vi "Get Autonomous Data.vi"(11 "Autonomous Selectin":string="Robot Right Switch Left") -> (3 "Autonomous Data Selected":T1(array[cluster]))   [LabVIEW 2017]
uses:
  Framework/Robot Global Data.vi
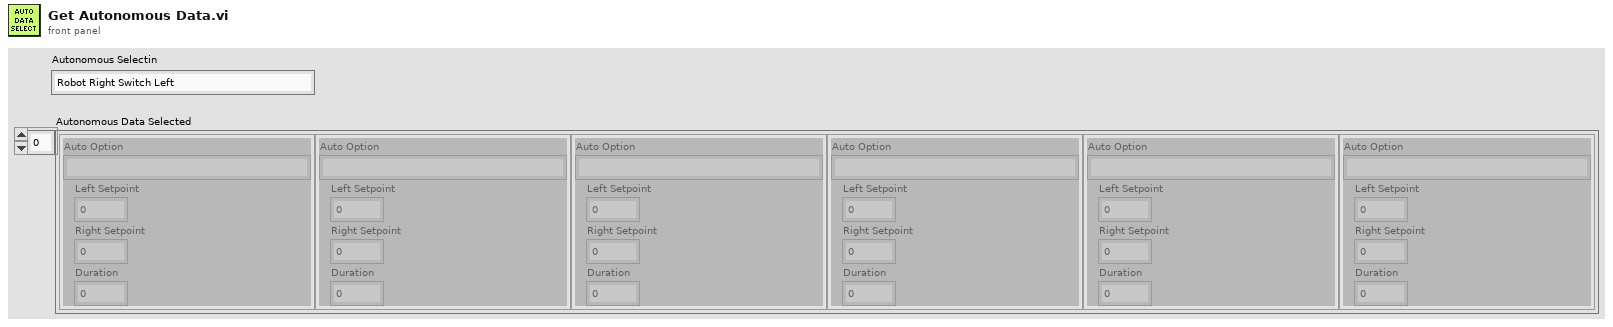
[diagram p1: front panel]
types:
  T1 = cluster{"Auto Option":string, "Left Setpoint":dbl, "Right Setpoint":dbl, "Duration":dbl}[]
  T2 = cluster{"Auto Option":string, "Left Setpoint":dbl, "Right Setpoint":dbl, "Duration":dbl}[][]
  T3 = cluster{"Auto Option":string, "Left Setpoint":dbl, "Right Setpoint":dbl, "Duration":dbl}
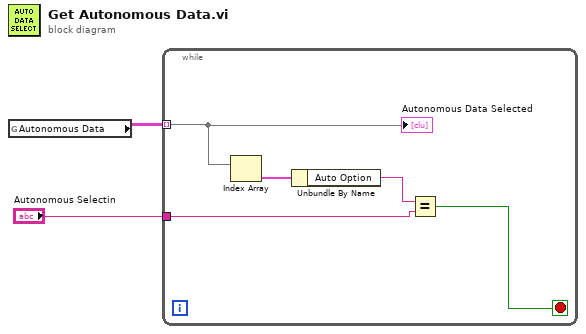
[diagram p0: block diagram]
diagram:
  n1 = global read "Robot Global Data.vi" "Autonomous Data"() -> (w1:T2)
  n2 = while {
    tunnel: w1 -> [w7] mode=indexing
    tunnel: "Autonomous Selectin" -> [w4]
    stop <- w3 stop-if-true
    n3 = Index Array(array=w7) -> (element=w6:T3)  [unwired: 1 in]
    n4 = Unbundle By Name(w6) -> ("Auto Option"=w5:string)
    n5 = Equal?(x=w5, y=w4) -> (x = y?=w3:bool)
    "Autonomous Data Selected" <- w7
  }
